vi "Powerup Clear.vi"(8 "error in (no error)":errorcluster, 11 "TCP Network Connection in":refnum<k5>) -> (0 "error out":errorcluster, 3 "connection ID out":refnum<k5>)   [LabVIEW 2024, in "OptoMMP.lvlib"]
doc: "Performs a PUC on the specified TCP network. \n\nThis action must be completed at device startup once a connection has been established. \"Powerup Clear\" must always be preceded by \"OptoMMP Open Connection\".\n\nLast updated: 8/6/2025"
uses:
  <instrlib>/OptoMMP/OptoMMP.lvlib
panel:
  # "Copyright (c) 2025 California Institute of Technology (Caltech).\nU.S. Government sponsorship acknowledged.\n\nLicensed under the Apache License, Version 2.0 (the \"License\");\nyou may not use this file except in compliance with the License.\nYou may obtain a copy of the License at\n\n    http://www.apache.org/licenses/LICENSE-2.0\n\nUnless required by applicable law or agreed to in writing, software\ndistributed under the License is distributed on an \"AS IS\" BASIS,\nWITHOUT WARRANTIES OR CONDITIONS OF ANY KIND, either express or implied.\nSee the License for the specific language governing permissions and\nlimitations under the License."
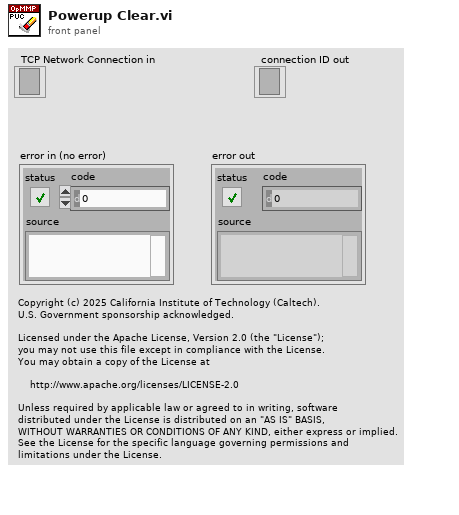
[diagram p1: front panel]
types:
  T1 = enum16{"Read Block Response", "Write Quadlet or Block Response", "Read Quadlet Response"}
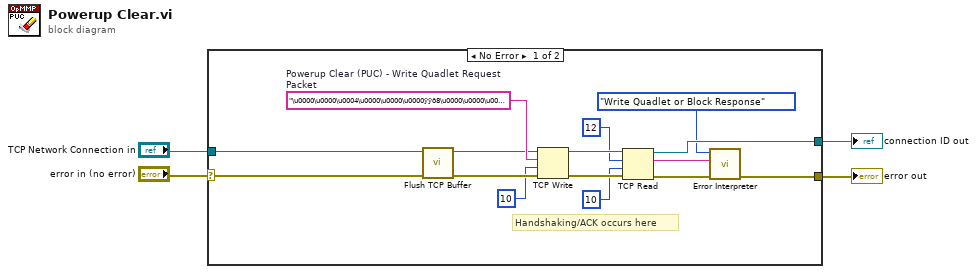
[diagram p0: block diagram]
diagram:
  n1 = case shown="No Error" "error in (no error)" {
    selector: "error in (no error)" -> [w8 w21]
    tunnel: [w14 w21] -> w4
    tunnel: [w12 w20] -> w3
    tunnel: "TCP Network Connection in" -> [w9 w20]
    frame No Error {
      w19 = "\u0000\u0000\u0004\u0000\u0000\u0000ÿÿð8\u0000\u0000\u0000\u0000\u0000\u0001"  # Powerup Clear (PUC) - Write Quadlet Request Packet
      # "Handshaking/ACK occurs here"
      n2 = call <instrlib>:"Flush TCP Buffer.vi"("error in (no error)"=w8, "TCP Network Connection in"=w9) -> ("error out"=w6:errorcluster, "TCP Network Connection out"=w7:refnum<k5>)  [unwired: 8 in]
      n3 = TCP Write(connection ID=w7, data in=w19, error in (no error)=w6, 9:10 ("timeout ms (25000)")) -> (connection ID out=w17:refnum<k5>, error out=w18:errorcluster)  [unwired: 1 out]
      n4 = TCP Read(connection ID=w17, bytes to read=12, error in (no error)=w18, 9:10 ("timeout ms (25000)")) -> (connection ID out=w12:refnum<k5>, data out=w11:string, error out=w15:errorcluster)  [unwired: 1 in]
      n5 = call <instrlib>:"Error Interpreter.vi"("error in (no error)"=w15, "data in"=w11, "packet type"=T1."Write Quadlet or Block Response") -> ("error out"=w14:errorcluster)  [unwired: 8 in]
    }
    frame Error {
    }
  }
  "error out" <- w4
  "connection ID out" <- w3
